vi "Connect_to_BSA_IP.vi"() -> (0 "error out":errorcluster, 1 "BSA":refnum<k7>)   [LabVIEW 2011]
uses:
  Globals/LDA_meas_global_1.vi
panel:
  in  "BSACtrl.IBSA":refnum<k7>
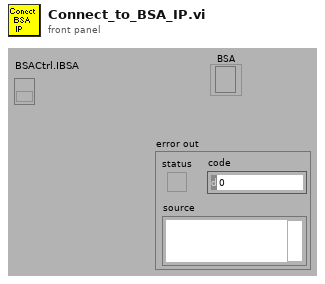
[diagram p1: front panel]
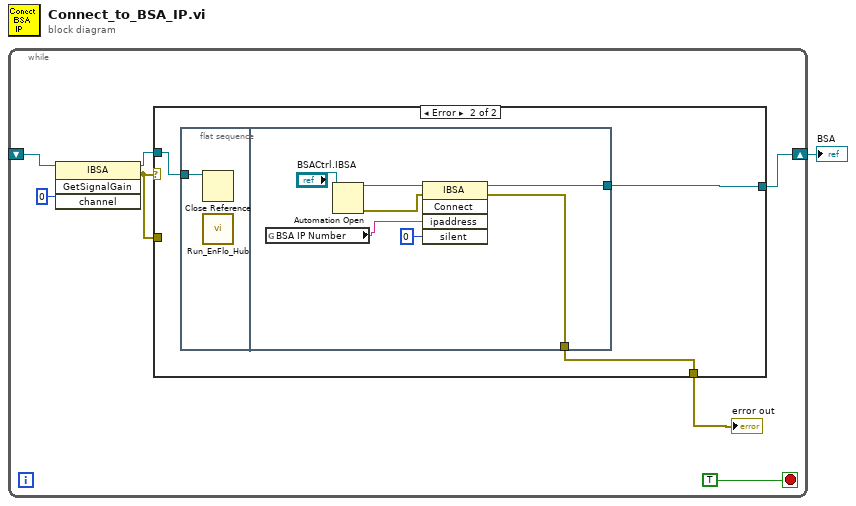
[diagram p0: block diagram]
diagram:
  n1 = while {
    shift-right: [w6] -> w1
    shift-left: _ -> [w7]
    stop <- TRUE stop-if-true
    n2 = invoke class="IBSA" method="GetSignalGain"(reference=w7, "channel"=0) -> (reference out=w5:refnum<k7>, error out=w2:errorcluster)  [unwired: 2 in, 2 out]
    n3 = case shown="Error" w2 {
      tunnel: [w10 w13] -> w6
      tunnel: w5 -> [w10 w11]
      tunnel: [w9 w12] -> w3
      tunnel: w2 -> [w9 _]
      frame No Error {
      }
      frame Error {
        n4 = flat-sequence {
          tunnel: w11 -> [w14]
          tunnel: [w16] -> w13
          tunnel: [w15] -> w12
          frame #0 {
            n5 = Close Reference(reference=w14) -> ()  [unwired: 1 in, 1 out]
            n6 = call "Run_EnFlo_Hub.vi"() -> ()  [unwired: 8 out]
          }
          frame #1 {
            n7 = global read "LDA_meas_global_1.vi" "BSA IP Number"() -> (w17:string)
            n8 = Automation Open(Automation Refnum="BSACtrl.IBSA") -> (Automation Refnum=w20:refnum<k7>, error out=w19:errorcluster)  [unwired: 2 in, 1 out]
            n9 = invoke class="IBSA" method="Connect"(reference=w20, error in=w19, "ipaddress"=w17, "silent"=0) -> (reference out=w16:refnum<k7>, error out=w15:errorcluster)  [unwired: 1 in, 3 out]
          }
        }
      }
    }
    "error out" <- w3
  }
  "BSA" <- w1
